vi "Get Control References.vi"(8 "error in (no error)":errorcluster, 9 "Controls to Exclude":refnum<vi>[](array[refnum]), 10 "VI Refnum":refnum<vi>, 11 "AbstractAutoRegistration in":refnum<class "AbstractAutoRegistration.lvclass">) -> (0 "error out":errorcluster, 2 "Controls":T1, 3 "AbstractAutoRegistration out":refnum<class "AbstractAutoRegistration.lvclass">)   [LabVIEW 2015, in "AutoRegistration.lvlib" / "AbstractAutoRegistration.lvclass"]
uses:
  AbstractAutoRegistration.lvclass
  Registration References.ctl
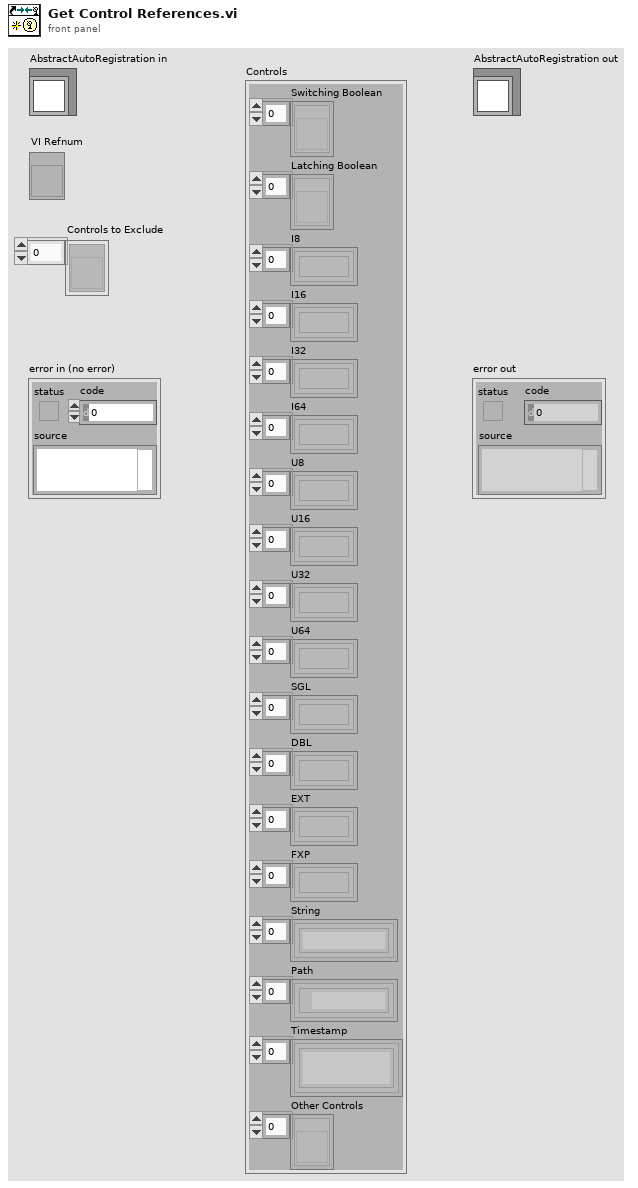
[diagram p1: front panel]
types:
  T1 = typedef "AutoRegistration.lvlib/AbstractAutoRegistration.lvclass/Registration References.ctl" = cluster{"Switching Boolean":refnum<vi>[], "Latching Boolean":refnum<vi>[], "I8":refnum<vi>[], "I16":refnum<vi>[], "I32":refnum<vi>[], "I64":refnum<vi>[], "U8":refnum<vi>[], "U16":refnum<vi>[], "U32":refnum<vi>[], "U64":refnum<vi>[], "SGL":refnum<vi>[], "DBL":refnum<vi>[], "EXT":refnum<vi>[], "FXP":refnum<vi>[], "String":refnum<vi>[], "Path":refnum<vi>[], "Timestamp":refnum<vi>[], "Other Controls":refnum<vi>[]}
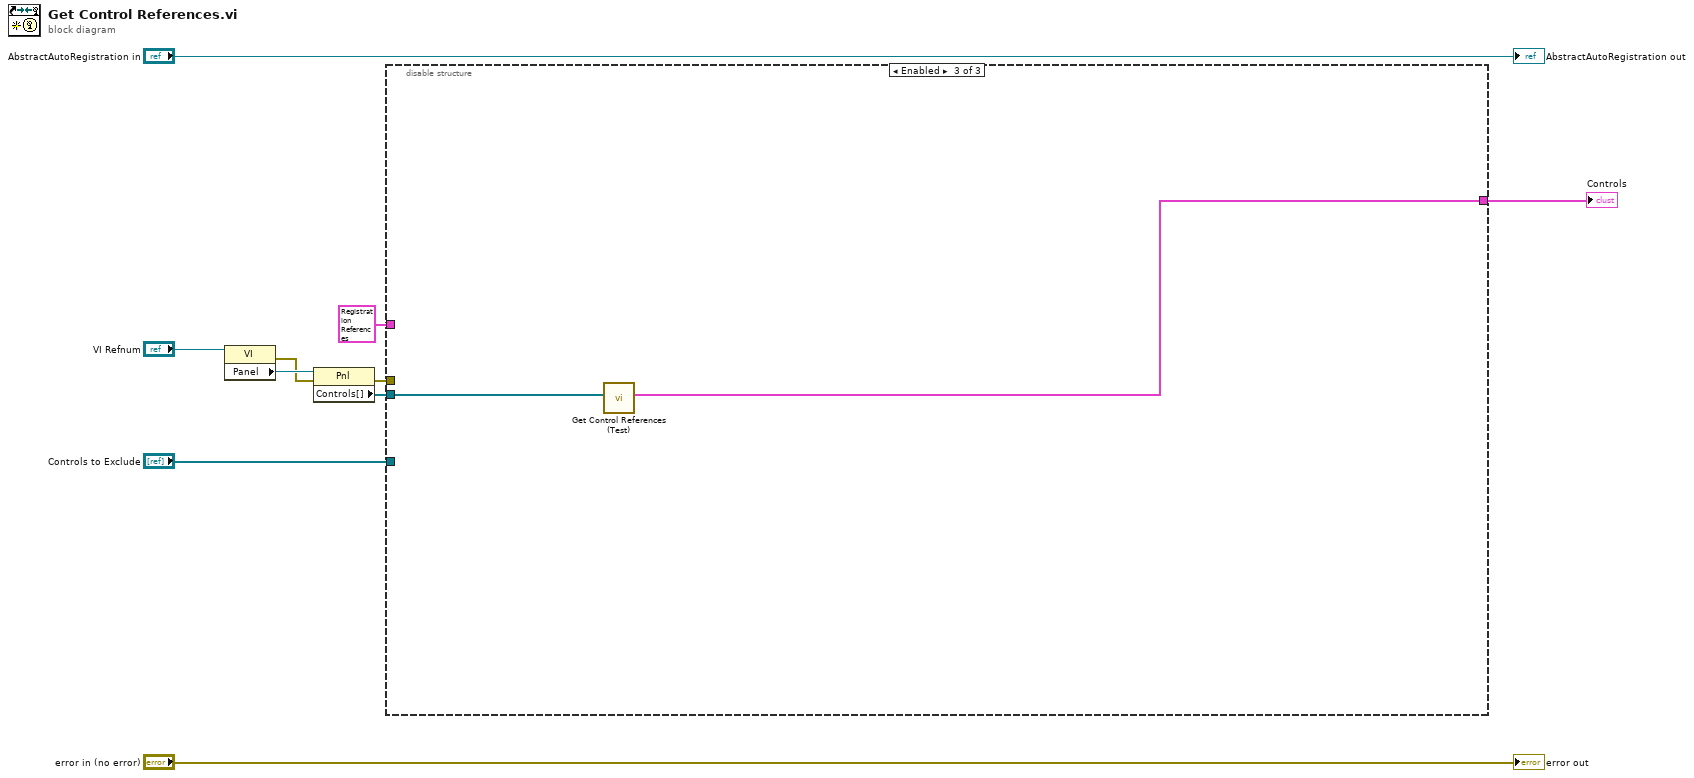
[diagram p0: block diagram]
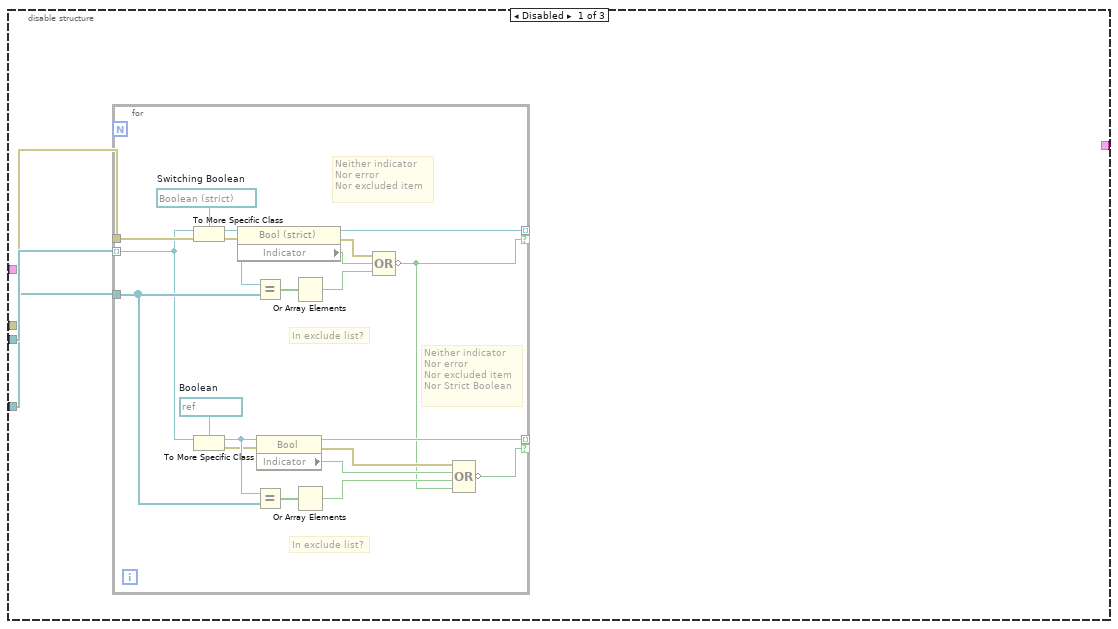
[diagram p2: hidden frame]
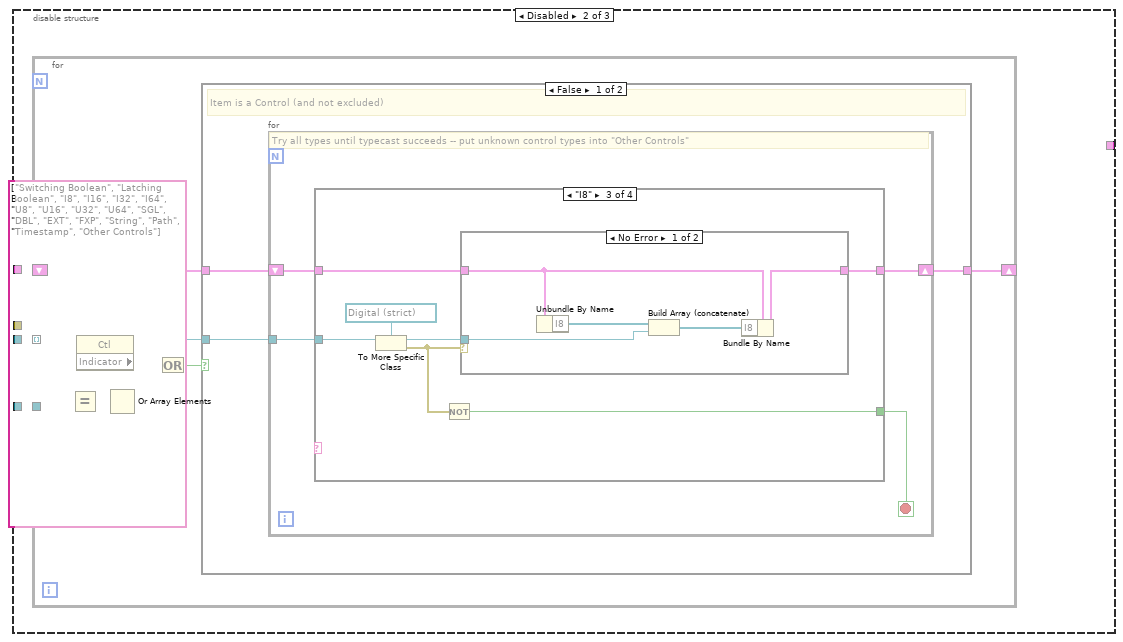
[diagram p3: hidden frame]
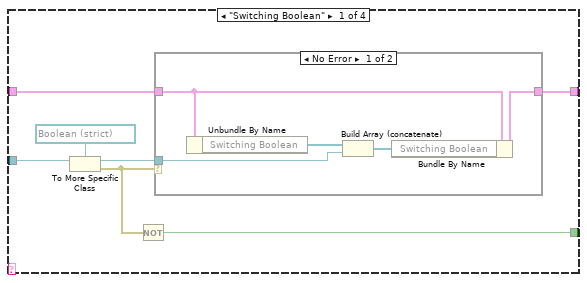
[diagram p4: hidden frame]
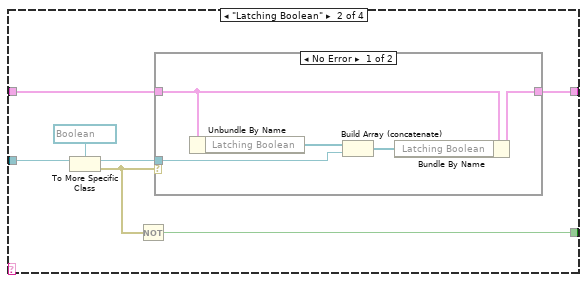
[diagram p6: hidden frame]
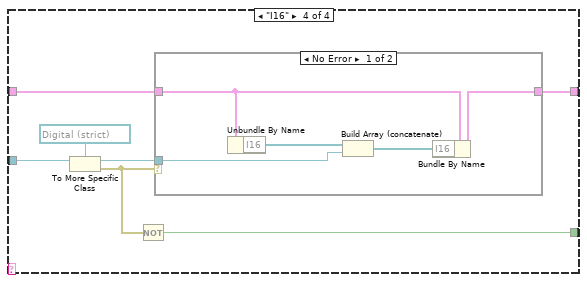
[diagram p9: hidden frame]
diagram:
  n1 = property class="VI"(reference="VI Refnum") -> (error out=w6:errorcluster, "Panel"=w7:refnum<vi>)  [unwired: 1 in, 1 out]
  n2 = property class="Pnl"(reference=w7, error in=w6) -> (error out=w4:errorcluster, "Controls[]"=w5:refnum<vi>[])  [unwired: 1 out]
  n3 = disable-structure shown="Enabled" {
    disable-tunnel: w5 -> [w15 w38 w110]
    disable-tunnel: w4 -> [w14 _ _]
    disable-tunnel: "Controls to Exclude" -> [w13 w39 _]
    disable-tunnel: T1 {"Switching Boolean"=[], "Latching Boolean"=[], "I8"=[], "I16"=[], "I32"=[], "I64"=[], "U8"=[], "U16"=[], "U32"=[], "U64"=[], "SGL"=[], "DBL"=[], "EXT"=[], "FXP"=[], "String"=[], "Path"=[], "Timestamp"=[], "Other Controls"=[]} ("Controls") -> [_ w37 _]
    disable-tunnel: [_ _ w109] -> w1
    frame Disabled {
      n4 = for {
        tunnel: w15 -> [w18] mode=indexing
        tunnel: w14 -> [w36]
        tunnel: w13 -> [w21]
        tunnel: [w35] -> w11 mode=indexing if=w19
        tunnel: [w24] -> w12 mode=indexing if=w23
        w16 = refnum<vi> refnum  # Boolean
        w17 = refnum<vi> refnum  # Switching Boolean
        # "Neither indicator\nNor error\nNor excluded item\nNor Strict Boolean"
        # "In exclude list?"
        # "Neither indicator\nNor error\nNor excluded item"
        # "In exclude list?"
        n5 = To More Specific Class(target class=w17, reference=w18, error in=w36) -> (specific class reference=w33:refnum<vi>, error out=w34:errorcluster)
        n6 = To More Specific Class(target class=w16, reference=w18) -> (specific class reference=w26:refnum<vi>, error out=w25:errorcluster)  [unwired: 1 in]
        n7 = property class="Bool (strict)"(reference=w33, error in=w34) -> (reference out=w35:refnum<vi>, error out=w31:errorcluster, "Indicator"=w32:bool)
        n8 = Equal?(x=w33, y=w21) -> (x = y?=w20:bool[])
        n9 = Equal?(x=w26, y=w21) -> (x = y?=w22:bool[])
        n10 = property class="Bool"(reference=w26, error in=w25) -> (reference out=w24:refnum<vi>, error out=w28:errorcluster, "Indicator"=w27:bool)
        n11 = Or Array Elements(Boolean array=w20) -> (logical OR=w30:bool)
        n12 = Or Array Elements(Boolean array=w22) -> (logical OR=w29:bool)
        n13 = Compound Arithmetic op=OR(w31, w32, w30) -> (invert w19:bool)
        n14 = Compound Arithmetic op=OR(w28, w27, w29, w19) -> (invert w23:bool)
      }
    }
    frame Disabled {
      (unwired) string[] ["Switching Boolean", "Latching Boolean", "I8", "I16", "I32", "I64", "U8", "U16", "U32", "U64", "SGL", "DBL", "EXT", "FXP", "String", "Path", "Timestamp", "Other Controls"] ("Array")
      n15 = for {
        tunnel: w39 -> [w45]
        tunnel: w38 -> [w44] mode=indexing
        shift-right: [w46] -> _
        shift-left: w37 -> [w47]
        n16 = Equal?(x=w44, y=w45) -> (x = y?=w43:bool[])
        n17 = property class="Ctl"(reference=w44) -> (reference out=w48:refnum<vi>, "Indicator"=w42:bool)  [unwired: 1 in, 1 out]
        n18 = Or Array Elements(Boolean array=w43) -> (logical OR=w41:bool)
        n19 = Or(x=w42, y=w41) -> (x .or. y?=w40:bool)
        n20 = case shown="False" w40 {
          tunnel: w48 -> [w49 _]
          tunnel: w47 -> [w51 w108]
          tunnel: [w50 w108] -> w46
          frame False {
            # "Item is a Control (and not excluded)"
            n21 = for {
              shift-right: [w54] -> w50
              shift-left: w51 -> [w55]
              tunnel: w49 -> [w53]
              stop <- w52 stop-if-true
              # "Try all types until typecast succeeds -- put unknown control types into \"Other Controls\""
              n22 = case shown="\"I8\"" {
                selector: _ -> [_ _ _ _]
                tunnel: w55 -> [w62 w75 w88 w101]
                tunnel: [w60 w73 w86 w99] -> w54
                tunnel: w53 -> [w61 w74 w87 w100]
                tunnel: [w56 w70 w83 w96] -> w52
                frame "Switching Boolean" {
                  n23 = To More Specific Class(target class=refnum<vi> refnum ("Switching Boolean"), reference=w61) -> (specific class reference=w59:refnum<vi>, error out=w57:errorcluster)  [unwired: 1 in]
                  n24 = Not(x=w57) -> (.not. x?=w56:bool)
                  n25 = case shown="No Error" w57 {
                    tunnel: w62 -> [w66 w68]
                    tunnel: [w67 w68] -> w60
                    tunnel: w59 -> [w64 _]
                    frame No Error {
                      n26 = Unbundle By Name(w66) -> ("Switching Boolean"=w65:refnum<vi>[])
                      n27 = Build Array (concatenate)(w65, w64) -> (w63:refnum<vi>[])
                      n28 = Bundle By Name(cluster=w66, "Switching Boolean"=w63) -> (w67:T1)
                    }
                    frame Error {
                    }
                  }
                }
                frame "Latching Boolean" {
                  n29 = To More Specific Class(target class=refnum<vi> refnum ("Latching Boolean"), reference=w74) -> (specific class reference=w72:refnum<vi>, error out=w71:errorcluster)  [unwired: 1 in]
                  n30 = Not(x=w71) -> (.not. x?=w70:bool)
                  n31 = case shown="No Error" w71 {
                    tunnel: w75 -> [w79 w81]
                    tunnel: [w80 w81] -> w73
                    tunnel: w72 -> [w77 _]
                    frame No Error {
                      n32 = Unbundle By Name(w79) -> ("Latching Boolean"=w78:refnum<vi>[])
                      n33 = Build Array (concatenate)(w78, w77) -> (w76:refnum<vi>[])
                      n34 = Bundle By Name(cluster=w79, "Latching Boolean"=w76) -> (w80:T1)
                    }
                    frame Error {
                    }
                  }
                }
                frame "I8" {
                  n35 = To More Specific Class(target class=refnum<vi> refnum ("I8"), reference=w87) -> (specific class reference=w85:refnum<vi>, error out=w84:errorcluster)  [unwired: 1 in]
                  n36 = Not(x=w84) -> (.not. x?=w83:bool)
                  n37 = case shown="No Error" w84 {
                    tunnel: w88 -> [w92 w94]
                    tunnel: [w93 w94] -> w86
                    tunnel: w85 -> [w90 _]
                    frame No Error {
                      n38 = Unbundle By Name(w92) -> ("I8"=w91:refnum<vi>[])
                      n39 = Build Array (concatenate)(w91, w90) -> (w89:refnum<vi>[])
                      n40 = Bundle By Name(cluster=w92, "I8"=w89) -> (w93:T1)
                    }
                    frame Error {
                    }
                  }
                }
                frame "I16" {
                  n41 = To More Specific Class(target class=refnum<vi> refnum ("I16"), reference=w100) -> (specific class reference=w98:refnum<vi>, error out=w97:errorcluster)  [unwired: 1 in]
                  n42 = Not(x=w97) -> (.not. x?=w96:bool)
                  n43 = case shown="No Error" w97 {
                    tunnel: w101 -> [w105 w107]
                    tunnel: [w106 w107] -> w99
                    tunnel: w98 -> [w103 _]
                    frame No Error {
                      n44 = Unbundle By Name(w105) -> ("I16"=w104:refnum<vi>[])
                      n45 = Build Array (concatenate)(w104, w103) -> (w102:refnum<vi>[])
                      n46 = Bundle By Name(cluster=w105, "I16"=w102) -> (w106:T1)
                    }
                    frame Error {
                    }
                  }
                }
              }
            }
          }
          frame True {
            # "Do nothing for indicators and excluded controls"
          }
        }
      }
    }
    frame Enabled {
      n47 = call "Get Control References (Test).vi"("Controls[]"=w110) -> ("Controls"=w109:T1)  [unwired: 10 in]
    }
  }
  "Controls" <- w1
  "error out" <- "error in (no error)"
  "AbstractAutoRegistration out" <- "AbstractAutoRegistration in"
